vi "Transfer_function_diagonal.vi"(0 "X reference":fxp<+/-,32,16>, 1 "Y reference":fxp<+/-,32,16>, 2 "Z reference":fxp<+/-,32,16>, 3 "X actual":fxp<+/-,33,17>, 4 "Y actual":fxp<+/-,33,17>, 5 "Z actual":fxp<+/-,33,17>, 6 "Scaling mV to V":fxp<+,33,10>=0.0009765625, 7 "xx1 Transfer Function":T1={"sos gain SF Controller"=0.0, "-a01(2)"=[0.0, 0.0, 0.0, 0.0, 0.0, 0.0, 0.0, 0.0, 0.0, 0.0, 0.0, 0.0, 0.0, 0.0, 0.0, 0.0, 0.0, 0.0, 0.0, 0.0], "-a02(2)"=[0.0, 0.0, 0.0, 0.0, 0.0, 0.0, 0.0, 0.0, 0.0, 0.0, 0.0, 0.0, 0.0, 0.0, 0.0, 0.0, 0.0, 0.0, 0.0, 0.0], "b01(2)"=[0.0, 0.0, 0.0, 0.0, 0.0, 0.0, 0.0, 0.0, 0.0, 0.0, 0.0, 0.0, 0.0, 0.0, 0.0, 0.0, 0.0, 0.0, 0.0, 0.0], "b02(2)"=[0.0, 0.0, 0.0, 0.0, 0.0, 0.0, 0.0, 0.0, 0.0, 0.0, 0.0, 0.0, 0.0, 0.0, 0.0, 0.0, 0.0, 0.0, 0.0, 0.0]}, 8 "Action":T2, 9 "yy1 Transfer Function":T1={"sos gain SF Controller"=0.0, "-a01(2)"=[0.0, 0.0, 0.0, 0.0, 0.0, 0.0, 0.0, 0.0, 0.0, 0.0, 0.0, 0.0, 0.0, 0.0, 0.0, 0.0, 0.0, 0.0, 0.0, 0.0], "-a02(2)"=[0.0, 0.0, 0.0, 0.0, 0.0, 0.0, 0.0, 0.0, 0.0, 0.0, 0.0, 0.0, 0.0, 0.0, 0.0, 0.0, 0.0, 0.0, 0.0, 0.0], "b01(2)"=[0.0, 0.0, 0.0, 0.0, 0.0, 0.0, 0.0, 0.0, 0.0, 0.0, 0.0, 0.0, 0.0, 0.0, 0.0, 0.0, 0.0, 0.0, 0.0, 0.0], "b02(2)"=[0.0, 0.0, 0.0, 0.0, 0.0, 0.0, 0.0, 0.0, 0.0, 0.0, 0.0, 0.0, 0.0, 0.0, 0.0, 0.0, 0.0, 0.0, 0.0, 0.0]}, 11 "zz1 Transfer Function":T1={"sos gain SF Controller"=0.0, "-a01(2)"=[0.0, 0.0, 0.0, 0.0, 0.0, 0.0, 0.0, 0.0, 0.0, 0.0, 0.0, 0.0, 0.0, 0.0, 0.0, 0.0, 0.0, 0.0, 0.0, 0.0], "-a02(2)"=[0.0, 0.0, 0.0, 0.0, 0.0, 0.0, 0.0, 0.0, 0.0, 0.0, 0.0, 0.0, 0.0, 0.0, 0.0, 0.0, 0.0, 0.0, 0.0, 0.0], "b01(2)"=[0.0, 0.0, 0.0, 0.0, 0.0, 0.0, 0.0, 0.0, 0.0, 0.0, 0.0, 0.0, 0.0, 0.0, 0.0, 0.0, 0.0, 0.0, 0.0, 0.0], "b02(2)"=[0.0, 0.0, 0.0, 0.0, 0.0, 0.0, 0.0, 0.0, 0.0, 0.0, 0.0, 0.0, 0.0, 0.0, 0.0, 0.0, 0.0, 0.0, 0.0, 0.0]}) -> (14 "X-stage voltage":fxp<+/-,32,16>, 15 "Y-stage voltage":fxp<+/-,32,16>, 16 "Z-stage voltage":fxp<+/-,32,16>, 17 "Kxx Output, Kxx*ex (V)":fxp<+/-,58,25>, 18 "Kyy Output, Kyy*ey (V)":fxp<+/-,58,25>, 19 "Kzz Output, Kzz*ez (V)":fxp<+/-,58,25>)   [LabVIEW 2015]
uses:
  Transfer_function_actions.ctl
  Transfer_function_coeffs.ctl
  <vilib>/rvi/Emulation/niFpgaGetClockAttributes.vi
  <vilib>/rvi/Emulation/niFpgaSctlEmulationGetInTimedLoop.vi
  <vilib>/rvi/Emulation/niFpgaEmulationReportErrorSimple.vi
  <vilib>/rvi/Emulation/niFpgaCriticalErrorInLSC.vi
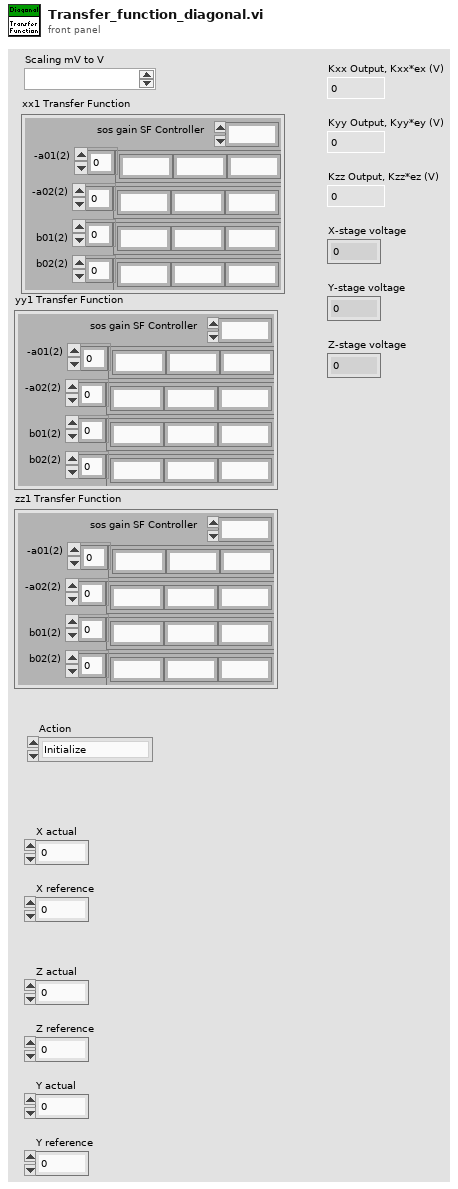
[diagram p1: front panel]
types:
  T1 = typedef "Transfer_function_coeffs.ctl" = cluster{"sos gain SF Controller":fxp<+/-,42,9>, "-a01(2)":fxp<+/-,64,9>[], "-a02(2)":fxp<+/-,64,9>[], "b01(2)":fxp<+/-,64,9>[], "b02(2)":fxp<+/-,64,9>[]}
  T2 = typedef "Transfer_function_actions.ctl" = enum16{"Initialize", "Calculate"}
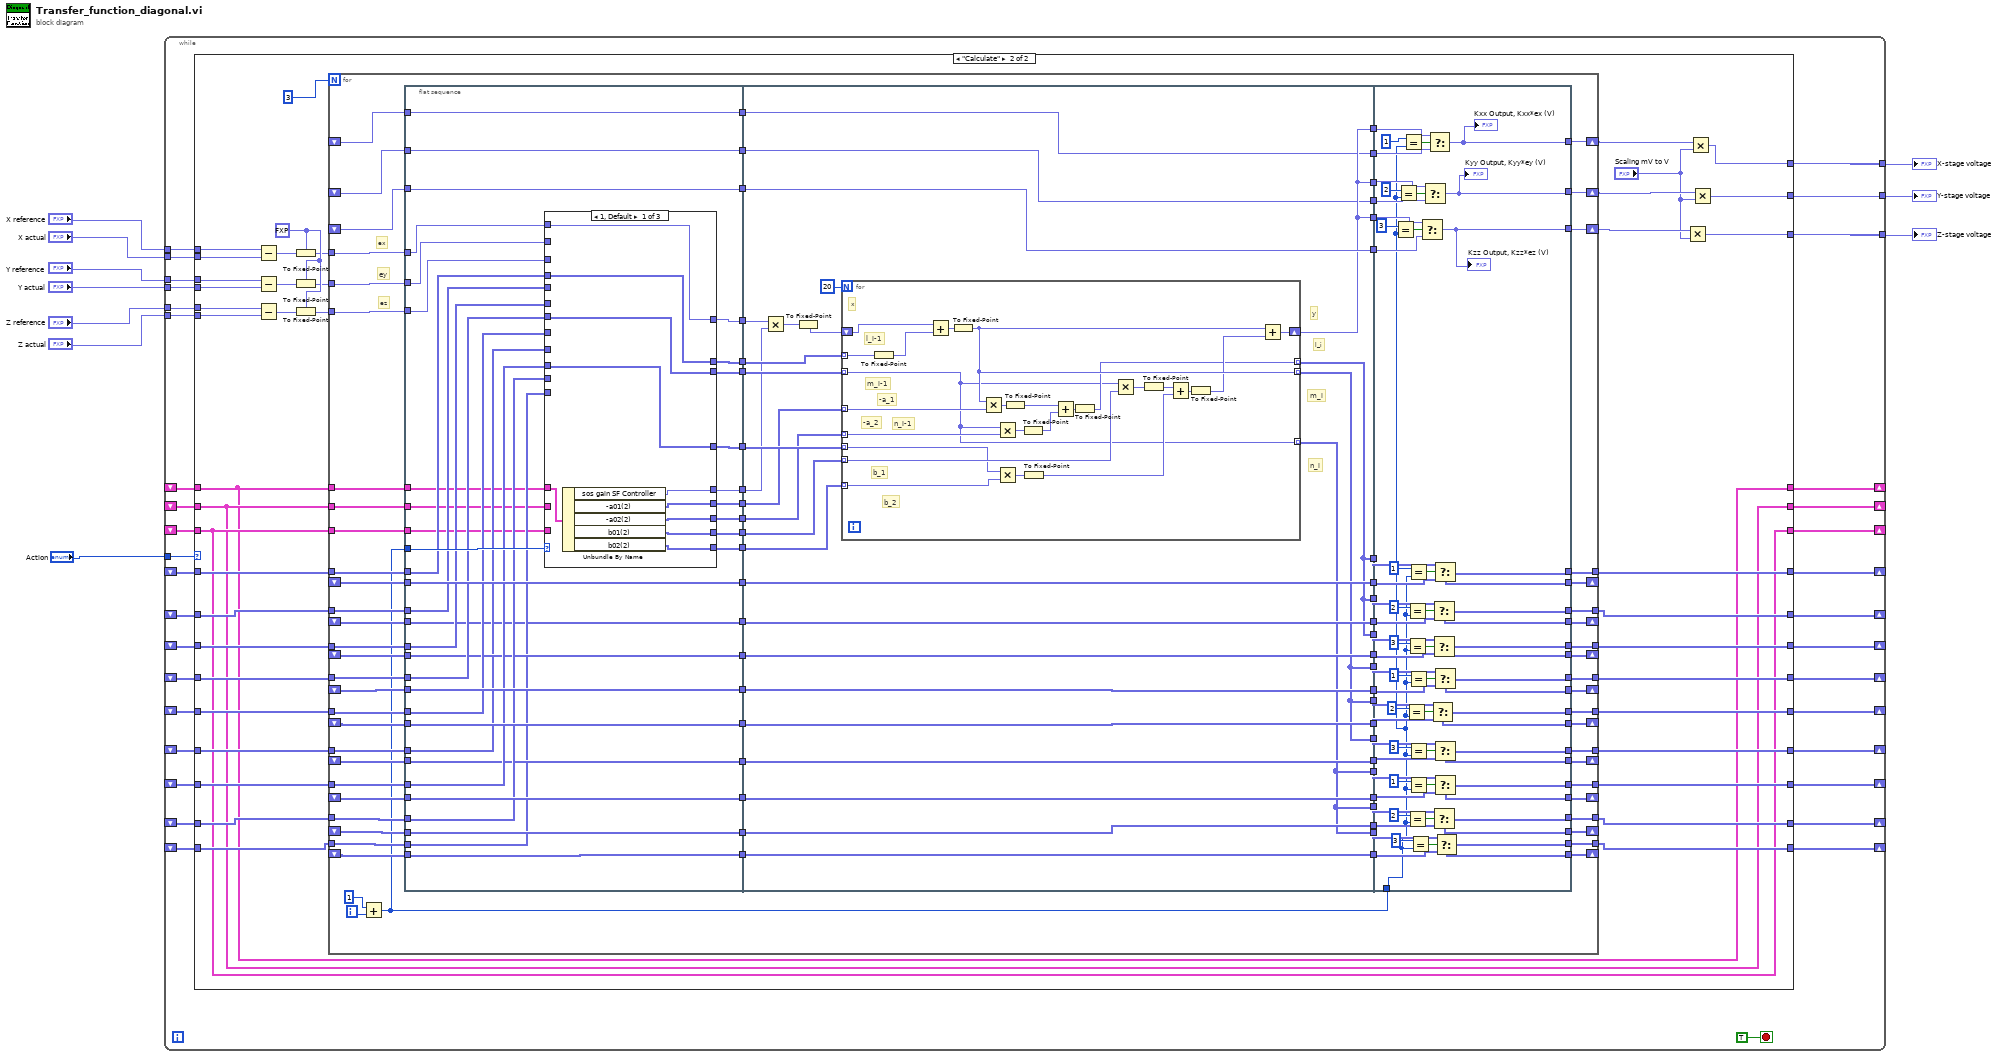
[diagram p0: block diagram]
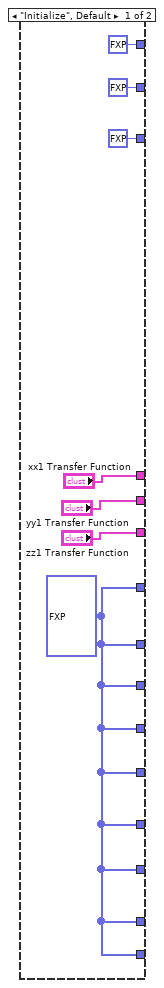
[diagram p2: hidden frame]
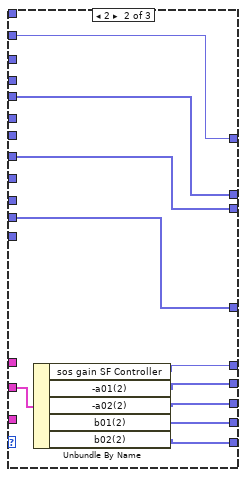
[diagram p3: hidden frame]
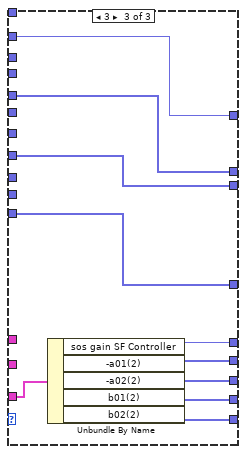
[diagram p4: hidden frame]
diagram:
  n1 = while {
    tunnel: [w45] -> w10
    tunnel: [w44] -> w9
    tunnel: [w43] -> w8
    tunnel: "Z reference" -> [w42]
    tunnel: "Y reference" -> [w41]
    tunnel: "X reference" -> [w40]
    tunnel: "Z actual" -> [w39]
    tunnel: "Y actual" -> [w38]
    tunnel: "X actual" -> [w37]
    shift-right: [w36] -> _
    shift-left: _ -> [w27]
    shift-right: [w29] -> _
    shift-left: _ -> [w20]
    shift-right: [w28] -> _
    shift-left: _ -> [w19]
    shift-right: [w35] -> _
    shift-left: _ -> [w26]
    shift-right: [w34] -> _
    shift-left: _ -> [w25]
    shift-right: [w33] -> _
    shift-left: _ -> [w24]
    shift-right: [w32] -> _
    shift-left: _ -> [w23]
    shift-right: [w31] -> _
    shift-left: _ -> [w22]
    shift-right: [w30] -> _
    shift-left: _ -> [w21]
    tunnel: "Action" -> [w17]
    shift-right: [w13] -> _
    shift-left: _ -> [w16]
    shift-right: [w12] -> _
    shift-left: _ -> [w15]
    shift-right: [w11] -> _
    shift-left: _ -> [w14]
    stop <- TRUE stop-if-true
    n2 = case shown="\"Calculate\"" w17 {
      tunnel: [fxp<+/-,32,16> 0.0 w94] -> w45
      tunnel: [fxp<+/-,32,16> 0.0 w93] -> w44
      tunnel: [fxp<+/-,32,16> 0.0 w92] -> w43
      tunnel: w42 -> [_ w91]
      tunnel: w41 -> [_ w90]
      tunnel: w40 -> [_ w89]
      tunnel: w39 -> [_ w82]
      tunnel: w38 -> [_ w80]
      tunnel: w37 -> [_ w79]
      tunnel: [w49 w73] -> w36
      tunnel: [w49 w72] -> w35
      tunnel: [w49 w71] -> w34
      tunnel: [w49 w70] -> w33
      tunnel: [w49 w69] -> w32
      tunnel: [w49 w68] -> w31
      tunnel: [w49 w67] -> w30
      tunnel: [w49 w66] -> w29
      tunnel: [w49 w65] -> w28
      tunnel: w27 -> [_ w64]
      tunnel: w26 -> [_ w63]
      tunnel: w25 -> [_ w62]
      tunnel: w24 -> [_ w61]
      tunnel: w23 -> [_ w60]
      tunnel: w22 -> [_ w59]
      tunnel: w21 -> [_ w58]
      tunnel: w20 -> [_ w57]
      tunnel: w19 -> [_ w56]
      tunnel: w16 -> [_ w53]
      tunnel: w15 -> [_ w54]
      tunnel: w14 -> [_ w55]
      tunnel: ["xx1 Transfer Function" w53] -> w13
      tunnel: ["yy1 Transfer Function" w54] -> w12
      tunnel: ["zz1 Transfer Function" w55] -> w11
      frame "Initialize", Default {
        w49 = fxp<+/-,58,25>[] [0.0, 0.0, 0.0, 0.0, 0.0, 0.0, 0.0, 0.0, 0.0, 0.0, 0.0, 0.0, 0.0, 0.0, 0.0, 0.0, 0.0, 0.0, 0.0, 0.0]
      }
      frame "Calculate" {
        w85 = fxp<+/-,58,25> 0.0 ("fixed-point type")
        n3 = Subtract(x=w89, y=w79) -> (x-y=w75:fxp<+/-,34,18>)
        n4 = Subtract(x=w90, y=w80) -> (x-y=w76:fxp<+/-,34,18>)
        n5 = Subtract(x=w91, y=w82) -> (x-y=w81:fxp<+/-,34,18>)
        n6 = To Fixed-Point(fixed-point type=w85, number=w75) -> (fixed-point=w77:fxp<+/-,58,25>)
        n7 = To Fixed-Point(fixed-point type=w85, number=w76) -> (fixed-point=w78:fxp<+/-,58,25>)
        n8 = To Fixed-Point(fixed-point type=w85, number=w81) -> (fixed-point=w83:fxp<+/-,58,25>)
        n9 = for {
          N: 3 -> [_]
          shift-right: [w175] -> w86
          shift-left: _ -> [w173]
          shift-right: [w172] -> w87
          shift-left: _ -> [w170]
          tunnel: [w163] -> w73
          shift-right: [w162] -> _
          shift-left: _ -> [w158]
          tunnel: [w161] -> w72
          shift-right: [w160] -> _
          shift-left: _ -> [w156]
          tunnel: w64 -> [w153]
          tunnel: w63 -> [w152]
          tunnel: [w151] -> w70
          shift-right: [w150] -> _
          shift-left: _ -> [w143]
          tunnel: [w149] -> w69
          shift-right: [w148] -> _
          shift-left: _ -> [w142]
          tunnel: [w147] -> w67
          tunnel: [w146] -> w66
          shift-right: [w145] -> _
          shift-left: _ -> [w141]
          shift-right: [w144] -> _
          shift-left: _ -> [w130]
          tunnel: w61 -> [w140]
          tunnel: w60 -> [w139]
          tunnel: w58 -> [w138]
          tunnel: w57 -> [w137]
          tunnel: w77 -> [w129]
          tunnel: w78 -> [w126]
          shift-right: [w125] -> w88
          shift-left: _ -> [w122]
          tunnel: [w117] -> w71
          tunnel: [w116] -> w68
          tunnel: [w115] -> w65
          shift-right: [w114] -> _
          shift-left: _ -> [w110]
          shift-right: [w113] -> _
          shift-left: _ -> [w108]
          shift-right: [w112] -> _
          shift-left: _ -> [w106]
          tunnel: w62 -> [w105]
          tunnel: w56 -> [w104]
          tunnel: w59 -> [w103]
          tunnel: w83 -> [w99]
          tunnel: w53 -> [w97]
          tunnel: w54 -> [w96]
          tunnel: w55 -> [w95]
          i -> [w180]
          # "ez"
          # "ey"
          # "ex"
          n10 = Add(x=1, y=w180) -> (x+y=w98:i32)
          n11 = flat-sequence {
            tunnel: [w226] -> w190
            tunnel: [w225] -> w189
            tunnel: [w224] -> w188
            tunnel: [w223] -> w187
            tunnel: [w222] -> w186
            tunnel: [w221] -> w185
            tunnel: [w220] -> w184
            tunnel: [w219] -> w183
            tunnel: w98 -> [w227]
            tunnel: [w205] -> w182
            tunnel: [w218] -> w174
            tunnel: w173 -> [w218]
            tunnel: [w217] -> w171
            tunnel: w170 -> [w217]
            tunnel: [w216] -> w159
            tunnel: w158 -> [w216]
            tunnel: [w197] -> w157
            tunnel: w156 -> [w197]
            tunnel: w153 -> [w207]
            tunnel: w152 -> [w208]
            tunnel: w143 -> [w215]
            tunnel: w142 -> [w214]
            tunnel: w141 -> [w213]
            tunnel: w140 -> [w209]
            tunnel: w139 -> [w210]
            tunnel: w138 -> [w211]
            tunnel: w137 -> [w212]
            tunnel: w130 -> [w206]
            tunnel: [w215] -> w136
            tunnel: [w214] -> w135
            tunnel: [w213] -> w134
            tunnel: w129 -> [w196]
            tunnel: [w206] -> w128
            tunnel: w126 -> [w195]
            tunnel: [w204] -> w123
            tunnel: w122 -> [w204]
            tunnel: [w203] -> w111
            tunnel: w110 -> [w203]
            tunnel: [w202] -> w109
            tunnel: w108 -> [w202]
            tunnel: [w201] -> w107
            tunnel: w106 -> [w201]
            tunnel: w105 -> [w198]
            tunnel: w104 -> [w200]
            tunnel: w103 -> [w199]
            tunnel: w99 -> [w194]
            tunnel: w97 -> [w193]
            tunnel: w96 -> [w192]
            tunnel: w95 -> [w191]
            tunnel: w190 -> [w283]
            tunnel: w189 -> [w282]
            tunnel: w188 -> [w281]
            tunnel: w187 -> [w261]
            tunnel: w186 -> [w262]
            tunnel: w185 -> [w263]
            tunnel: w184 -> [w264]
            tunnel: w183 -> [w265]
            tunnel: w182 -> [w270]
            tunnel: [w268] -> w179
            tunnel: [w268] -> w178
            tunnel: [w259] -> w177
            tunnel: [w260] -> w176
            tunnel: w174 -> [w260]
            tunnel: w171 -> [w259]
            tunnel: [w269] -> w169
            tunnel: [w269] -> w168
            tunnel: [w267] -> w167
            tunnel: [w267] -> w166
            tunnel: [w266] -> w165
            tunnel: [w266] -> w164
            tunnel: w159 -> [w280]
            tunnel: w157 -> [w279]
            tunnel: [w280] -> w155
            tunnel: [w279] -> w154
            tunnel: w136 -> [w278]
            tunnel: w135 -> [w277]
            tunnel: w134 -> [w276]
            tunnel: [w278] -> w133
            tunnel: [w277] -> w132
            tunnel: [w276] -> w131
            tunnel: w128 -> [w275]
            tunnel: [w275] -> w127
            tunnel: [w268] -> w124
            tunnel: w123 -> [w274]
            tunnel: [w274] -> w121
            tunnel: [w269] -> w120
            tunnel: [w267] -> w119
            tunnel: [w266] -> w118
            tunnel: w111 -> [w273]
            tunnel: w109 -> [w272]
            tunnel: w107 -> [w271]
            tunnel: [w273] -> w102
            tunnel: [w272] -> w101
            tunnel: [w271] -> w100
            tunnel: w179 -> [w311]
            tunnel: w178 -> [w366]
            tunnel: w98 -> [w310]
            tunnel: w177 -> [w365]
            tunnel: w176 -> [w312]
            tunnel: [w315] -> w175
            tunnel: [w314] -> w172
            tunnel: w169 -> [w352]
            tunnel: w168 -> [w351]
            tunnel: w167 -> [w350]
            tunnel: w166 -> [w349]
            tunnel: w165 -> [w348]
            tunnel: w164 -> [w347]
            tunnel: [w346] -> w163
            tunnel: [w346] -> w162
            tunnel: [w345] -> w161
            tunnel: [w345] -> w160
            tunnel: w155 -> [w344]
            tunnel: w154 -> [w343]
            tunnel: [w342] -> w151
            tunnel: [w342] -> w150
            tunnel: [w341] -> w149
            tunnel: [w341] -> w148
            tunnel: [w340] -> w147
            tunnel: [w339] -> w146
            tunnel: [w340] -> w145
            tunnel: [w339] -> w144
            tunnel: w133 -> [w338]
            tunnel: w132 -> [w337]
            tunnel: w131 -> [w336]
            tunnel: w127 -> [w335]
            tunnel: [w313] -> w125
            tunnel: w124 -> [w332]
            tunnel: w121 -> [w331]
            tunnel: w120 -> [w324]
            tunnel: w119 -> [w323]
            tunnel: w118 -> [w322]
            tunnel: [w321] -> w117
            tunnel: [w320] -> w116
            tunnel: [w319] -> w115
            tunnel: [w321] -> w114
            tunnel: [w320] -> w113
            tunnel: [w319] -> w112
            tunnel: w102 -> [w318]
            tunnel: w101 -> [w317]
            tunnel: w100 -> [w316]
            frame #0 {
              n12 = case shown="1, Default" w227 {
                tunnel: [w233 w242 w252] -> w223
                tunnel: [w232 w241 w251] -> w222
                tunnel: [w231 w240 w250] -> w221
                tunnel: [w230 w239 w249] -> w220
                tunnel: [w229 w238 w248] -> w219
                tunnel: [w234 w246 w256] -> w224
                tunnel: [w235 w245 w255] -> w225
                tunnel: [w236 w244 w254] -> w226
                tunnel: w207 -> [w236 _ _]
                tunnel: w208 -> [_ w244 _]
                tunnel: w209 -> [w235 _ _]
                tunnel: w210 -> [_ w245 _]
                tunnel: w211 -> [w234 _ _]
                tunnel: w212 -> [_ w246 _]
                tunnel: [w237 w247 w257] -> w205
                tunnel: w196 -> [w237 _ _]
                tunnel: w195 -> [_ w247 _]
                tunnel: w200 -> [_ _ w256]
                tunnel: w199 -> [_ _ w255]
                tunnel: w198 -> [_ _ w254]
                tunnel: w194 -> [_ _ w257]
                tunnel: w193 -> [w228 _ _]
                tunnel: w192 -> [_ w243 _]
                tunnel: w191 -> [_ _ w253]
                frame 1, Default {
                  n13 = Unbundle By Name(w228) -> ("sos gain SF Controller"=w233:fxp<+/-,42,9>, "-a01(2)"=w232:fxp<+/-,64,9>[], "-a02(2)"=w231:fxp<+/-,64,9>[], "b01(2)"=w230:fxp<+/-,64,9>[], "b02(2)"=w229:fxp<+/-,64,9>[])
                }
                frame 2 {
                  n14 = Unbundle By Name(w243) -> ("sos gain SF Controller"=w242:fxp<+/-,42,9>, "-a01(2)"=w241:fxp<+/-,64,9>[], "-a02(2)"=w240:fxp<+/-,64,9>[], "b01(2)"=w239:fxp<+/-,64,9>[], "b02(2)"=w238:fxp<+/-,64,9>[])
                }
                frame 3 {
                  n15 = Unbundle By Name(w253) -> ("sos gain SF Controller"=w252:fxp<+/-,42,9>, "-a01(2)"=w251:fxp<+/-,64,9>[], "-a02(2)"=w250:fxp<+/-,64,9>[], "b01(2)"=w249:fxp<+/-,64,9>[], "b02(2)"=w248:fxp<+/-,64,9>[])
                }
              }
            }
            frame #1 {
              # "n_i"
              # "m_i"
              # "l_i"
              # "y"
              n16 = Multiply(x=w270, y=w261) -> (x*y=w284:fxp<+/-,64,34>)
              n17 = To Fixed-Point(number=w284) -> (fixed-point=w285:fxp<+/-,58,25>)  [unwired: 1 in]
              n18 = for {
                N: 20 -> [_]
                tunnel: w262 -> [w302] mode=indexing
                tunnel: w265 -> [w299] mode=indexing
                shift-right: [w304] -> w268
                shift-left: w285 -> [w303]
                tunnel: w263 -> [w301] mode=indexing
                tunnel: w264 -> [w300] mode=indexing
                tunnel: [w291] -> w269 mode=indexing
                tunnel: w283 -> [w297] mode=indexing
                tunnel: [w294] -> w267 mode=indexing
                tunnel: w282 -> [w287] mode=indexing
                tunnel: [w287] -> w266 mode=indexing
                tunnel: w281 -> [w295] mode=indexing
                # "b_1"
                # "b_2"
                # "n_i-1"
                # "-a_2"
                # "-a_1"
                # "m_i-1"
                # "l_i-1"
                # "x"
                n19 = To Fixed-Point(number=w297) -> (fixed-point=w309:fxp<+/-,58,25>)  [unwired: 1 in]
                n20 = Add(x=w303, y=w309) -> (x+y=w296:fxp<+/-,59,26>)
                n21 = To Fixed-Point(number=w296) -> (fixed-point=w294:fxp<+/-,58,25>)  [unwired: 1 in]
                n22 = Multiply(x=w294, y=w302) -> (x*y=w286:fxp<+/-,64,34>)
                n23 = Multiply(x=w295, y=w299) -> (x*y=w308:fxp<+/-,64,34>)
                n24 = Multiply(x=w287, y=w301) -> (x*y=w305:fxp<+/-,64,34>)
                n25 = To Fixed-Point(number=w286) -> (fixed-point=w290:fxp<+/-,58,25>)  [unwired: 1 in]
                n26 = To Fixed-Point(number=w305) -> (fixed-point=w289:fxp<+/-,58,25>)  [unwired: 1 in]
                n27 = To Fixed-Point(number=w308) -> (fixed-point=w288:fxp<+/-,58,25>)  [unwired: 1 in]
                n28 = Add(x=w290, y=w289) -> (x+y=w298:fxp<+/-,59,26>)
                n29 = To Fixed-Point(number=w298) -> (fixed-point=w291:fxp<+/-,58,25>)  [unwired: 1 in]
                n30 = Multiply(x=w287, y=w300) -> (x*y=w306:fxp<+/-,64,34>)
                n31 = To Fixed-Point(number=w306) -> (fixed-point=w292:fxp<+/-,58,25>)  [unwired: 1 in]
                n32 = Add(x=w292, y=w288) -> (x+y=w307:fxp<+/-,59,26>)
                n33 = To Fixed-Point(number=w307) -> (fixed-point=w293:fxp<+/-,58,25>)  [unwired: 1 in]
                n34 = Add(x=w294, y=w293) -> (x+y=w304:fxp<+/-,58,25>)
              }
            }
            frame #2 {
              n35 = Equal?(x=3, y=w310) -> (x = y?=w333:bool)
              n36 = Equal?(x=2, y=w310) -> (x = y?=w367:bool)
              n37 = Equal?(x=1, y=w310) -> (x = y?=w369:bool)
              n38 = Equal?(x=2, y=w310) -> (x = y?=w357:bool)
              n39 = Equal?(x=2, y=w310) -> (x = y?=w361:bool)
              n40 = Equal?(x=3, y=w310) -> (x = y?=w329:bool)
              n41 = Equal?(x=2, y=w310) -> (x = y?=w353:bool)
              n42 = Equal?(x=1, y=w310) -> (x = y?=w363:bool)
              n43 = Equal?(x=1, y=w310) -> (x = y?=w359:bool)
              n44 = Equal?(x=3, y=w310) -> (x = y?=w327:bool)
              n45 = Equal?(x=1, y=w310) -> (x = y?=w355:bool)
              n46 = Equal?(x=3, y=w310) -> (x = y?=w325:bool)
              n47 = Select(t=w332, s=w333, f=w331) -> (s? t:f=w313:fxp<+/-,58,25>)
              "Kzz Output, Kzz*ez (V)" <- w313
              n48 = Select(t=w366, s=w367, f=w365) -> (s? t:f=w314:fxp<+/-,58,25>)
              "Kyy Output, Kyy*ey (V)" <- w314
              n49 = Select(t=w311, s=w369, f=w312) -> (s? t:f=w315:fxp<+/-,58,25>)
              "Kxx Output, Kxx*ex (V)" <- w315
              n50 = Select(t=w349, s=w357, f=w337) -> (s? t:f=w341:fxp<+/-,58,25>[])
              n51 = Select(t=w351, s=w361, f=w343) -> (s? t:f=w345:fxp<+/-,58,25>[])
              n52 = Select(t=w324, s=w329, f=w318) -> (s? t:f=w321:fxp<+/-,58,25>[])
              n53 = Select(t=w347, s=w353, f=w335) -> (s? t:f=w339:fxp<+/-,58,25>[])
              n54 = Select(t=w352, s=w363, f=w344) -> (s? t:f=w346:fxp<+/-,58,25>[])
              n55 = Select(t=w350, s=w359, f=w338) -> (s? t:f=w342:fxp<+/-,58,25>[])
              n56 = Select(t=w323, s=w327, f=w317) -> (s? t:f=w320:fxp<+/-,58,25>[])
              n57 = Select(t=w348, s=w355, f=w336) -> (s? t:f=w340:fxp<+/-,58,25>[])
              n58 = Select(t=w322, s=w325, f=w316) -> (s? t:f=w319:fxp<+/-,58,25>[])
            }
          }
        }
        n59 = Multiply(x=w88, y="Scaling mV to V") -> (x*y=w93:fxp<+/-,32,16>)
        n60 = Multiply(x=w86, y="Scaling mV to V") -> (x*y=w94:fxp<+/-,32,16>)
        n61 = Multiply(x=w87, y="Scaling mV to V") -> (x*y=w92:fxp<+/-,32,16>)
      }
    }
  }
  "X-stage voltage" <- w10
  "Z-stage voltage" <- w9
  "Y-stage voltage" <- w8
